vi "Stepper Mover Act.vi"(0 "command text in":string[](array[string])) -> ()   [LabVIEW 2021]
uses:
  VI Server Control N1/VI Server Control.ctl
panel:
  out "String":string
  in  "VI Server Control":T1={"VI name"="", "Control"=[], "Value"=[], "Boolean?"=[], "Control to End"="", "Condition"=enum."within xxx% of target value", "xxx%"=0.0, "Target Value"=0.0, "Timeout (sec)"=120.0, "wait (sec)"=120.0, "check every (s)"=120.0, "Boolean indi"=FALSE} {"Boolean?" min=0.0 max=1.0 step=1.0 format="%#_1g"}
  # "0"
  # "1"
  # "2"
  # "3"
  # "4"
  # "5"
  # "6"
  # "7"
  # "8"
  # "9"
  # "Finish if"
  # "is"
  # "and also finish the whole thing if time elapses"
  # "or longer."
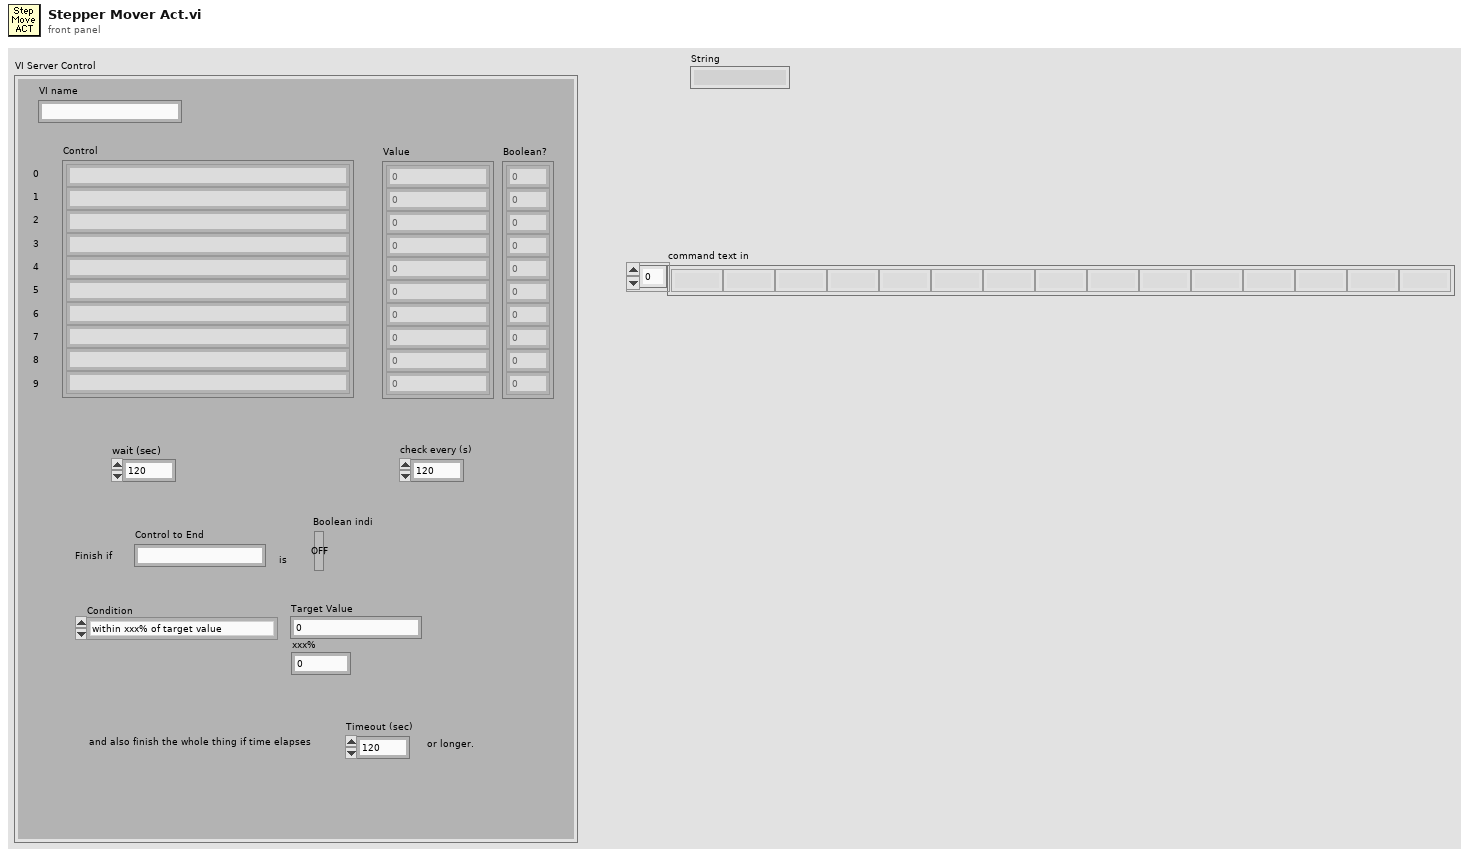
[diagram p1: front panel]
types:
  T1 = typedef "VI Server Control.ctl" = cluster{"VI name":string, "Control":string[], "Value":dbl[], "Boolean?":dbl[], "Control to End":string, "Condition":enum16{"within xxx% of target value", "<= target value", ">= target value", "= target value"}, "xxx%":dbl, "Target Value":dbl, "Timeout (sec)":dbl, "wait (sec)":dbl, "check every (s)":dbl, "Boolean indi":bool}
  T2 = typedef "Stepper Mover.ctl" = cluster{"extra wait":i32, "Stepper Value":dbl, "Top or Bottom":enum32{"Move to Top Position (deg)", "Move to Bottom Position (deg or in)"}}
  T3 = enum16{"within xxx% of target value", "<= target value", ">= target value", "= target value"}
  T4 = enum32{"Move to Top Position (deg)", "Move to Bottom Position (deg or in)"}
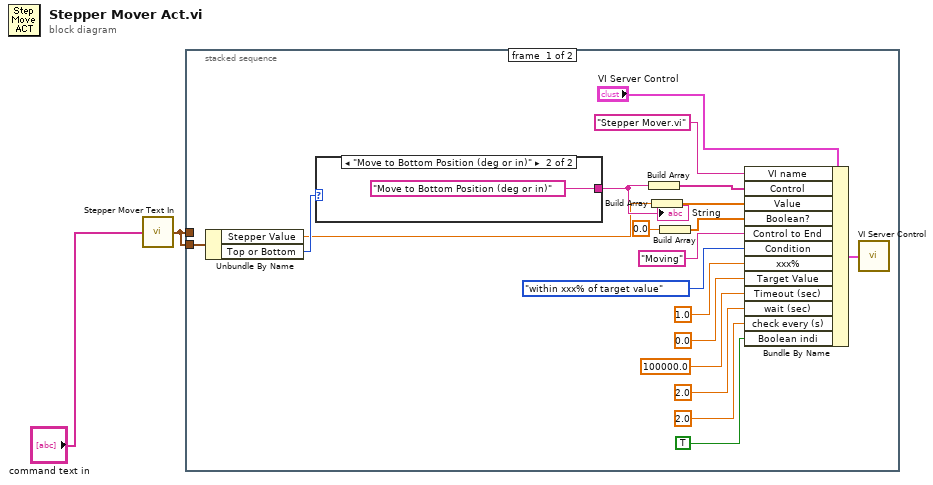
[diagram p0: block diagram]
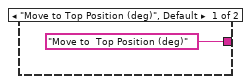
[diagram p2: hidden frame]
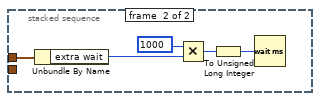
[diagram p3: hidden frame]
diagram:
  n1 = call "Stepper Mover Text In.vi"("command text in"="command text in") -> ("Stepper Mover"=w2:T2)
  n2 = stacked-sequence {
    tunnel: w2 -> [w21 _]
    tunnel: w2 -> [_ w25]
    frame #0 {
      n3 = Unbundle By Name(w21) -> ("Stepper Value"=w14:dbl, "Top or Bottom"=w17:T4)
      n4 = case shown="\"Move to Bottom Position (deg or in)\"" w17 {
        tunnel: ["Move to  Top Position (deg)" "Move to Bottom Position (deg or in)"] -> w15
        frame "Move to Top Position (deg)", Default {
        }
        frame "Move to Bottom Position (deg or in)" {
        }
      }
      "String" <- w15
      n5 = Build Array(w15) -> (w16:string[])
      n6 = Build Array(w14) -> (w13:dbl[])
      n7 = Build Array(0.0 ("element")) -> (w12:dbl[])
      n8 = Bundle By Name(cluster="VI Server Control", "VI name"="Stepper Mover.vi", "Control"=w16, "Value"=w13, "Boolean?"=w12, "Control to End"="Moving", "Condition"=T3."within xxx% of target value", "xxx%"=1.0, "Target Value"=0.0, "Timeout (sec)"=100000.0, "wait (sec)"=2.0, "check every (s)"=2.0, "Boolean indi"=TRUE) -> (w20:T1)
      n9 = call "VI Server Control.vi"("VI Server Control"=w20) -> ()
    }
    frame #1 {
      n10 = Unbundle By Name(w25) -> ("extra wait"=w24:i32)
      n11 = Multiply(x=1000 ("y"), y=w24) -> (x*y=w27:i32)
      n12 = To Unsigned Long Integer(number=w27) -> (unsigned 32bit integer=w26:u32)
      n13 = Wait (ms)(milliseconds to wait=w26) -> ()  [unwired: 1 out]
    }
  }
